vi "createViewer.vi"(7 "CommandEvents.lvclass":refnum<class "CommandEvents.lvclass">, 8 "error in (no error)":errorcluster, 9 "SettingsEventsManager.lvclass":refnum<class "SettingsEventsManager.lvclass">, 10 "Path":path, 11 "Tools.lvlib:Settings.lvlib:SettingsViewer.lvclass":refnum<class "settingsViewer.lvclass">) -> (0 "error out":errorcluster, 3 "SettingsViewer out":refnum<class "settingsViewer.lvclass">)   [LabVIEW 2011, in "Views.lvlib" / "SettingsViewer.lvclass"]
uses:
  settingsViewer.lvclass
  SettingsEventManager/SettingsEventsManager.lvclass
  CommandProcessor/CommandEvents/CommandEvents.lvclass
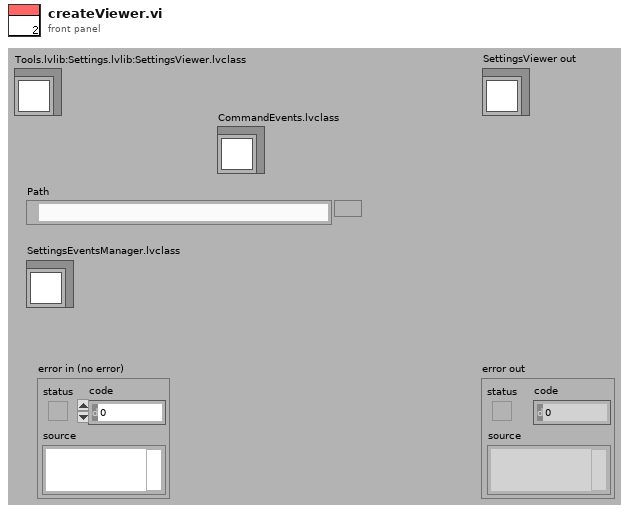
[diagram p1: front panel]
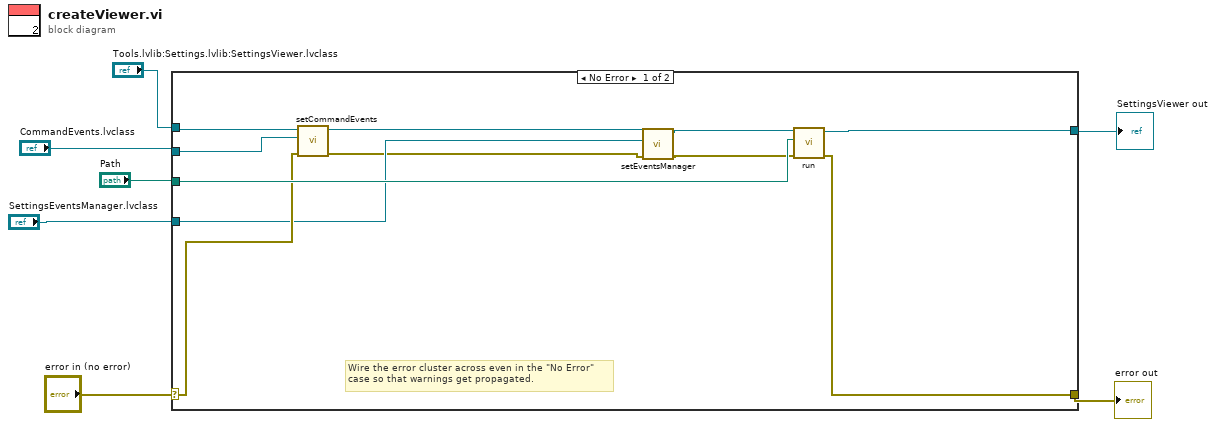
[diagram p0: block diagram]
diagram:
  n1 = case shown="No Error" "error in (no error)" {
    selector: "error in (no error)" -> [w14 w20]
    tunnel: [w10 w20] -> w6
    tunnel: [w17 w19] -> w5
    tunnel: "SettingsEventsManager.lvclass" -> [w12 _]
    tunnel: "Path" -> [w18 _]
    tunnel: "Tools.lvlib:Settings.lvlib:SettingsViewer.lvclass" -> [w16 w19]
    tunnel: "CommandEvents.lvclass" -> [w13 _]
    frame No Error {
      # "Wire the error cluster across even in the \"No Error\"\ncase so that warnings get propagated."
      n2 = call-dynamic "setCommandEvents.vi"("error in (no error)"=w14, "CommandEvents.lvclass"=w13, "SettingsViewer.lvclass in"=w16) -> ("error out"=w11:errorcluster, "SettingsViewer.lvclass out"=w15:refnum<class "settingsViewer.lvclass">)  [unwired: 7 in]
      n3 = call-dynamic "setEventsManager.vi"("error in (no error)"=w11, "Tools.lvlib:Settings.lvlib:SettingsEventsManager.lvclass"=w12, "settingsViewer.lvclass in"=w15) -> ("error out"=w8:errorcluster, "settingsViewer.lvclass out"=w9:refnum<class "settingsViewer.lvclass">)  [unwired: 7 in]
      n4 = call-dynamic "run.vi"("error in (no error)"=w8, "Path"=w18, "settingsViewer in"=w9) -> ("error out"=w10:errorcluster, "settingsViewer out"=w17:refnum<class "settingsViewer.lvclass">)  [unwired: 7 in]
    }
    frame Error {
    }
  }
  "error out" <- w6
  "SettingsViewer out" <- w5
